vi "더하기.vi"() -> ()   [LabVIEW 2014]
panel:
  out "출력 변수":dbl
  in  "입력 변수 2":dbl
  in  "입력 변수":dbl
  out "A 7":dbl
  in  "N":dbl
  out "A 6":dbl
  in  "A 5":dbl
  in  "A 4":dbl
  in  "A 3":dbl
  in  "A 2":dbl
  in  "A":dbl
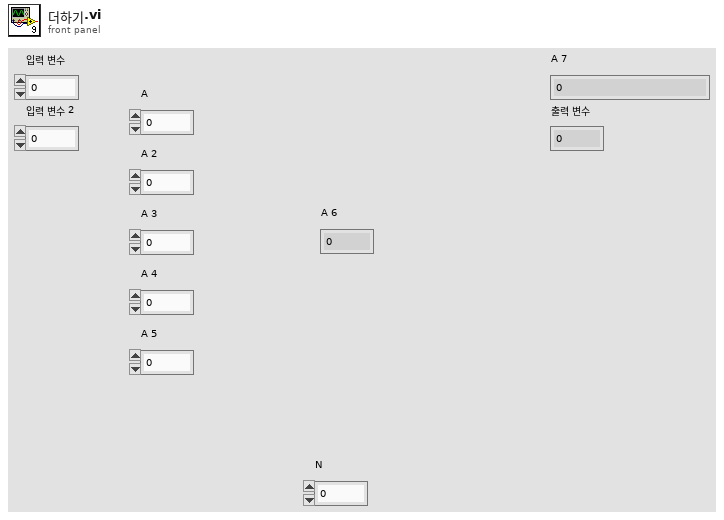
[diagram p1: front panel]
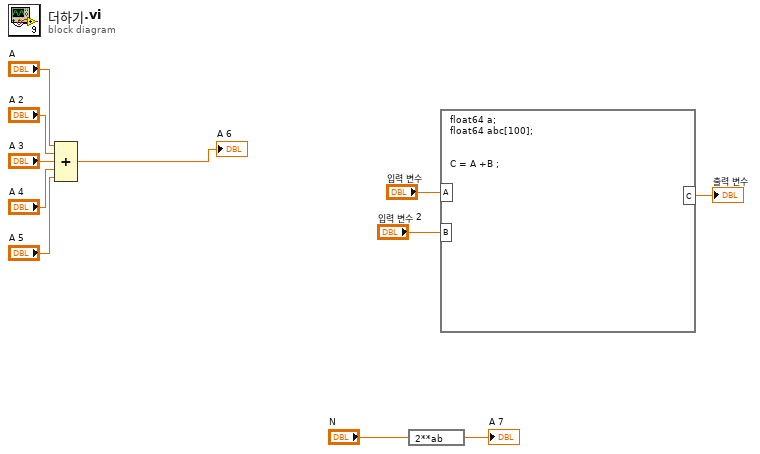
[diagram p0: block diagram]
diagram:
  n1 = Compound Arithmetic op=ADD("A", "A 2", "A 3", "A 4", "A 5") -> (→"A 6":dbl)
  n2 = expression code="2**ab"("N") -> (→"A 7":dbl)
  n3 = formula code="float64 a;\nfloat64 abc[100];\n\n\nC = A +B ;"("A"="입력 변수", "B"="입력 변수 2") -> ("C"=→"출력 변수":dbl)
